vi "Measure.vi"(8 "error in (no error)":errorcluster, 9 "measurement configuration":variant, 10 "measure call context in":refnum<class "Measure Call Context.lvclass">, 11 "measurement plugin in":refnum<class "Automotive Vision.lvclass">) -> (0 "error out":errorcluster, 1 "measurement results":variant, 2 "measure call context out":refnum<class "Measure Call Context.lvclass">, 3 "measurement plugin out":refnum<class "Automotive Vision.lvclass">)   [LabVIEW 2025, in "Automotive Vision.lvclass"]
uses:
  Automotive Vision.lvclass
  <vilib>/Plug-In SDKs/Measurements/Measure Call Context/Measure Call Context.lvclass
  Measurement Configuration.ctl
  Automotive Vision.lvclass/Automotive Vision.ctl
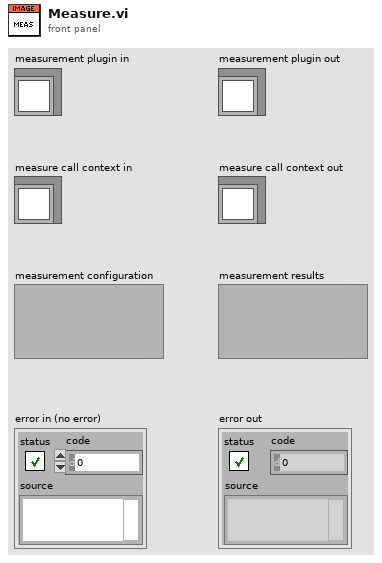
[diagram p1: front panel]
types:
  T1 = typedef "Automotive Vision.lvclass/Measurement Configuration.ctl" = cluster{"SERIAL (SI) CHANNEL":string, "PATH TO CONFIGURATION SCRIPT":string, "REF. CLOCK  (Hz)":dbl, "POC SOURCE":u32, "CSI-2 DATA SOURCE":u32, "SI ACTIVE LANE COUNT":u32, "PAYLOAD DATA TYPE":enum32{"Frame Start", "Frame End", "Line Start", "Line End", "End of Transmission", "Reserved 0", "Reserved 1", "Reserved 2", "Generic Short Packet 1", "Generic Short Packet 2", "Generic Short Packet 3", "Generic Short Packet 4", "Generic Short Packet 5", "Generic Short Packet 6", "Generic Short Packet 7", "Generic Short Packet 8", "Null", "Blanking Data", "Embedded 8-bit non Image Data", "Generic Long Packet 1", "Generic Long Packet 2", "Generic Long Packet 3", "Generic Long Packet 4", "Reserved 3", "YUV420 8-bit", "YUV420 10-bit", "Legacy YUV420 8-bit", "Reserved 4", "YUV420 8-bit Chroma Shifted", "YUV420 10-bit Chroma Shifted", "YUV422 8-bit", "YUV422 10-bit", "RGB444", "RGB555", "RGB565", "RGB666", "RGB888", "Reserved 5", "Reserved 6", "RAW 24", "RAW 6", "RAW 7", "RAW 8", "RAW 10", "RAW 12", "RAW 14", "RAW 16", "RAW 20", "User Defined 8-bit Data 1", "User Defined 8-bit Data 2", "User Defined 8-bit Data 3", "User Defined 8-bit Data 4", "User Defined 8-bit Data 5", "User Defined 8-bit Data 6", "User Defined 8-bit Data 7", "User Defined 8-bit Data 8", "USL Command", "Reserved 7", "Reserved 8", "Reserved 9", "Reserved 10", "Reserved 11", "Reserved 12", "LRTE EPD Spacer"}, "INTERPRETATION":u32, "VIRTUAL CHANNEL":u32, "PATTERN":u32, "ALGORITHM":u32}
  T2 = typedef "Automotive Vision.lvclass/Measurement Results.ctl" = cluster{"ACQ. IN PROGRESS":bool, "Array":u32[], "ACQ. DURATION (s)":dbl, "SOURCE RATE (fps)":dbl, "BYTES ACQUIRED":u64, "FRAME COUNT":u64, "POC VOLTAGE (V)":dbl, "POC CURRENT (A)":dbl, "ERROR":bool, "STATE MESSAGE":string, "IMAGE DATA":string}
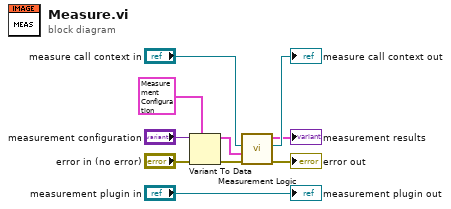
[diagram p0: block diagram]
diagram:
  n1 = Variant To Data(error in="error in (no error)", type=T1 {"SERIAL (SI) CHANNEL"="Lorem ipsum dolor sit", "PATH TO CONFIGURATION SCRIPT"="", "REF. CLOCK  (Hz)"=1.2, "POC SOURCE"=32, "CSI-2 DATA SOURCE"=64, "SI ACTIVE LANE COUNT"=64, "PAYLOAD DATA TYPE"=enum."Frame Start", "INTERPRETATION"=4294967264, "VIRTUAL CHANNEL"=4294967232, "PATTERN"=4294967232, "ALGORITHM"=1} ("measurement configuration"), Variant="measurement configuration") -> (data=w2:T1, error out=w7:errorcluster)
  n2 = call "Measurement Logic.vi"("error in"=w7, "measurement configuration"=w2, "measure call context in"="measure call context in") -> ("Error Out"=→"error out":errorcluster, "measure call context out"=→"measure call context out":refnum<class "Measure Call Context.lvclass">, "measurement results"=→"measurement results":T2)  [unwired: 6 in]
  "measurement plugin out" <- "measurement plugin in"
